vi "forward_dist_calc.vi"(0 "dt":dbl, 2 "Sodar Past":dbl, 3 "Forward Right":dbl, 4 "Sodar":dbl, 5 "Forward Left Past":dbl, 6 "Forward Left":dbl, 7 "Forward Right Past":dbl) -> (1 "Forward distance":dbl)   [LabVIEW 2015]
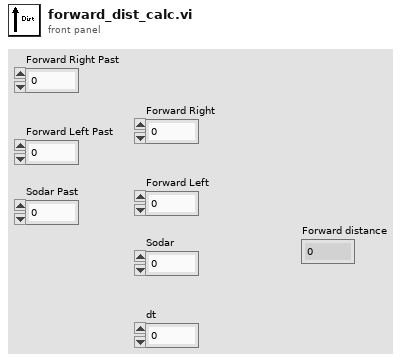
[diagram p1: front panel]
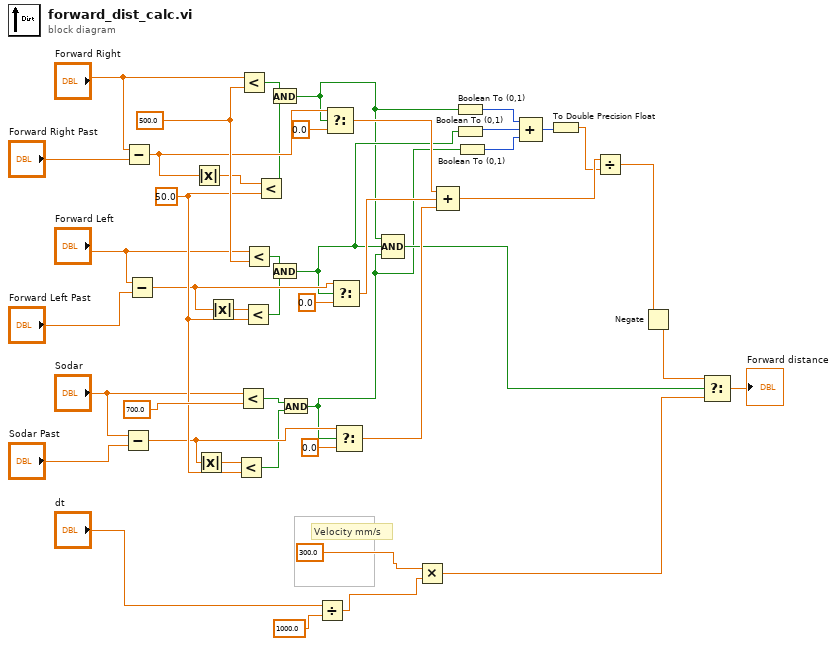
[diagram p0: block diagram]
diagram:
  w21 = 50.0 ("y")
  w45 = 500.0
  # "Velocity mm/s"
  n1 = Subtract(x="Sodar", y="Sodar Past") -> (x-y=w19:dbl)
  n2 = Subtract(x="Forward Right", y="Forward Right Past") -> (x-y=w22:dbl)
  n3 = Subtract(x="Forward Left", y="Forward Left Past") -> (x-y=w20:dbl)
  n4 = Absolute Value(x=w22) -> (abs(x)=w9:dbl)
  n5 = Absolute Value(x=w19) -> (abs(x)=w7:dbl)
  n6 = Absolute Value(x=w20) -> (abs(x)=w8:dbl)
  n7 = Less?(x=w7, y=w21) -> (x < y?=w17:bool)
  n8 = Less?(x="Sodar", y=700.0) -> (x < y?=w18:bool)
  n9 = Less?(x="Forward Right", y=w45) -> (x < y?=w12:bool)
  n10 = Less?(x=w8, y=w21) -> (x < y?=w14:bool)
  n11 = Less?(x="Forward Left", y=w45) -> (x < y?=w15:bool)
  n12 = Less?(x=w9, y=w21) -> (x < y?=w11:bool)
  n13 = And(x=w12, y=w11) -> (x .and. y?=w10:bool)
  n14 = And(x=w15, y=w14) -> (x .and. y?=w13:bool)
  n15 = And(x=w18, y=w17) -> (x .and. y?=w16:bool)
  n16 = Divide(x="dt", y=1000.0) -> (x/y=w23:dbl)
  n17 = Select(t=w22, s=w10, f=0.0) -> (s? t:f=w36:dbl)
  n18 = Select(t=w20, s=w13, f=0.0) -> (s? t:f=w35:dbl)
  n19 = Select(t=w19, s=w16, f=0.0) -> (s? t:f=w34:dbl)
  n20 = Compound Arithmetic op=AND(w10, w13, w16) -> (w27:bool)
  n21 = Multiply(x=300.0, y=w23) -> (x*y=w26:dbl)
  n22 = Compound Arithmetic op=ADD(w36, w35, w34) -> (w29:dbl)
  n23 = Boolean To (0,1)(Boolean=w10) -> (0, 1=w33:i16)
  n24 = Boolean To (0,1)(Boolean=w13) -> (0, 1=w32:i16)
  n25 = Boolean To (0,1)(Boolean=w16) -> (0, 1=w31:i16)
  n26 = Compound Arithmetic op=ADD(w33, w32, w31) -> (w30:i16)
  n27 = To Double Precision Float(number=w30) -> (double precision float=w28:dbl)
  n28 = Divide(x=w29, y=w28) -> (x/y=w3:dbl)
  n29 = Negate(x=w3) -> (-x=w1:dbl)
  n30 = Select(t=w1, s=w27, f=w26) -> (s? t:f=→"Forward distance":dbl)
